vi "PC Host.vi"() -> ()   [LabVIEW 2015]
panel:
  out "Resolution 2":u16
  in  "Resolution":u16(ring)=512 items=["2048*2048"=2048, "1024*1024"=1024, "512*512"=512, "256*256"=256]
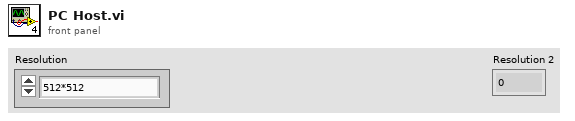
[diagram p1: front panel]
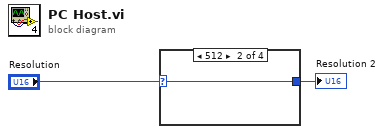
[diagram p0: block diagram]
diagram:
  n1 = case shown="512" "Resolution" {
    selector: "Resolution" -> [w3 w4 w5 w6]
    tunnel: [w3 w4 w5 w6] -> w1
    frame 256, Default {
    }
    frame 512 {
    }
    frame 1024 {
    }
    frame 2048 {
    }
  }
  "Resolution 2" <- w1
